vi "Radau5_Estimate Derivative Y.vi"(10 "Stage Y'":dbl[][](array[numeric]), 11 "Old Y'":dbl[](array[numeric])) -> (3 "Estimate Y' out":dbl[](array[numeric]))   [LabVIEW 2020, in "NI_DAE.lvlib"]
uses:
  <vilib>/gmath/NI_DAE.lvlib
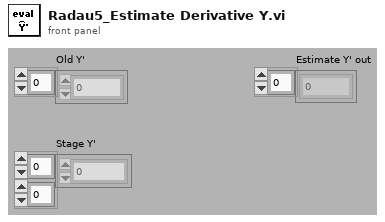
[diagram p1: front panel]
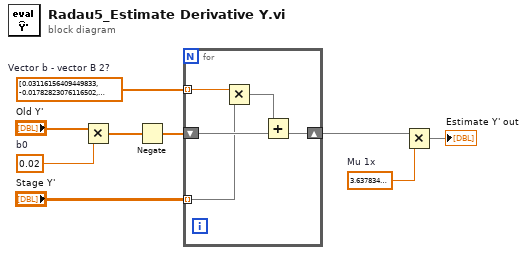
[diagram p0: block diagram]
diagram:
  w1 = 3.637834252744496  # Mu 1x
  w2 = dbl[] [0.03116156409449833, -0.01782823076116502, 0.2815566666666667]  # Vector b - vector B 2?
  w4 = 0.02  # b0
  n1 = Multiply(x="Old Y'", y=w4) -> (x*y=w8:dbl[])
  n2 = Negate(x=w8) -> (-x=w7:dbl[])
  n3 = for {
    tunnel: "Stage Y'" -> [w11] mode=indexing
    shift-right: [w13] -> w6
    shift-left: w7 -> [w14]
    tunnel: w2 -> [w10] mode=indexing
    n4 = Multiply(x=w10, y=w11) -> (x*y=w12:dbl[])
    n5 = Add(x=w12, y=w14) -> (x+y=w13:dbl[])
  }
  n6 = Multiply(x=w6, y=w1) -> (x*y=→"Estimate Y' out":dbl[])
